vi "Detach.vi"(0 "reference in":refnum<class "Subject.lvclass">, 1 "ObServer.lvclass":refnum<class "ObServer.lvclass">, 5 "error in (no error)":errorcluster) -> (14 "reference out":refnum<class "Subject.lvclass">, 19 "error out":errorcluster)   [LabVIEW 2013, in "Subject.lvclass"]
uses:
  Subject.lvclass
  ObServer_class/ObServer.lvclass
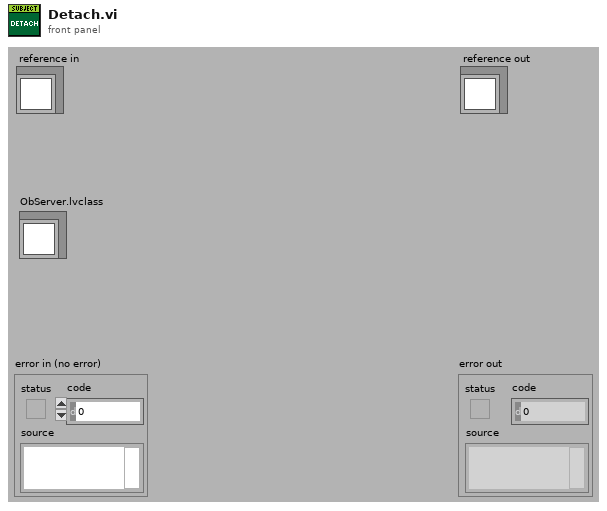
[diagram p1: front panel]
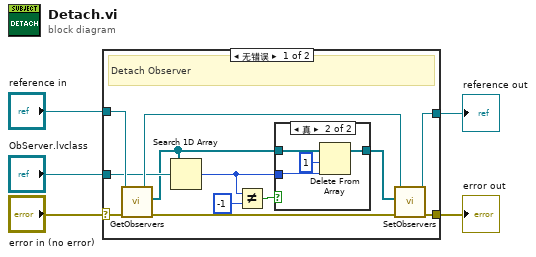
[diagram p0: block diagram]
diagram:
  n1 = case shown="无错误" "error in (no error)" {
    selector: "error in (no error)" -> [w8 w24]
    tunnel: [w6 w24] -> w4
    tunnel: [w15 w23] -> w2
    tunnel: "reference in" -> [w17 w23]
    tunnel: "ObServer.lvclass" -> [w14 _]
    frame No Error {
      # "Detach Observer"
      n2 = call-dynamic "GetObservers.vi"("error in (no error)"=w8, "reference in"=w17) -> ("error out"=w7:errorcluster, "Observers"=w11:refnum<class "ObServer.lvclass">[], "reference out"=w16:refnum<class "Subject.lvclass">)  [unwired: 7 in]
      n3 = Search 1D Array(1D array=w11, element=w14) -> (index of element=w10:i32)  [unwired: 1 in]
      n4 = Not Equal?(x=w10, y=-1) -> (x != y?=w12:bool)
      n5 = case shown="真" w12 {
        tunnel: w11 -> [w18 w22]
        tunnel: w10 -> [_ w21]
        tunnel: [w18 w19] -> w9
        frame False {
        }
        frame True {
          n6 = Delete From Array(array=w22, length=1 ("长度"), index=w21) -> (array with subset deleted=w19:refnum<class "ObServer.lvclass">[])  [unwired: 1 out]
        }
      }
      n7 = call-dynamic "SetObservers.vi"("error in (no error)"=w7, "Observers"=w9, "reference in"=w16) -> ("error out"=w6:errorcluster, "reference out"=w15:refnum<class "Subject.lvclass">)  [unwired: 7 in]
    }
    frame Error {
    }
  }
  "error out" <- w4
  "reference out" <- w2
